vi "createNotifiers.vi"(8 "error in":errorcluster) -> (0 "error out":errorcluster, 3 "notifiers":T1)   [LabVIEW 2017, in "notifiers.lvlib"]
uses:
  notifiers.lvlib
  notifiers.ctl
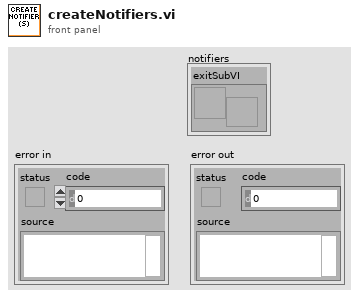
[diagram p1: front panel]
types:
  T1 = typedef "notifiers.lvlib/notifiers.ctl" = cluster{"exitSubVI":refnum<notifier>}
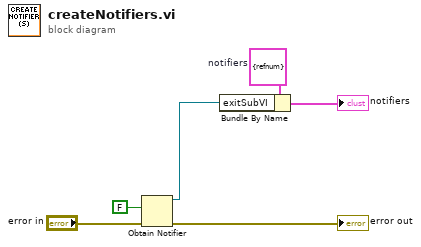
[diagram p0: block diagram]
diagram:
  w2 = T1 {"exitSubVI"=refnum}  # notifiers
  n1 = Obtain Notifier(notification data type=FALSE, error in (no error)="error in") -> (notifier out=w4:refnum<notifier>, error out=→"error out":errorcluster)  [unwired: 2 in, 1 out]
  n2 = Bundle By Name(cluster=w2, "exitSubVI"=w4) -> (→"notifiers":T1)
